vi "Compare_Connections_Disconnections.vi"(9 "VI_Disconnections":u8[](array[numeric]), 10 "VI_Connections":u8[](array[numeric]), 11 "Numeric":i32) -> (3 "Boolean":bool)   [LabVIEW 2014]
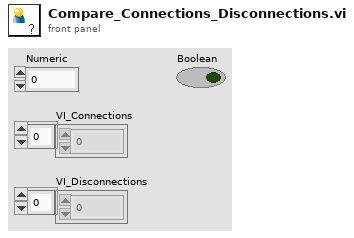
[diagram p1: front panel]
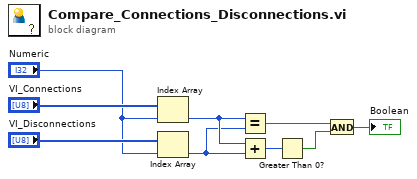
[diagram p0: block diagram]
diagram:
  n1 = Index Array(array="VI_Connections", index="Numeric") -> (element=w8:u8)
  n2 = Index Array(array="VI_Disconnections", index="Numeric") -> (element=w7:u8)
  n3 = Equal?(x=w8, y=w7) -> (x = y?=w2:bool)
  n4 = Add(x=w8, y=w7) -> (x+y=w4:u8)
  n5 = Greater Than 0?(x=w4) -> (x > 0?=w3:bool)
  n6 = And(x=w2, y=w3) -> (x .and. y?=→"Boolean":bool)
